vi "Create Coverage Report - With Custom Time Stamp - Reports Same Time.vi"() -> ()   [LabVIEW 2017, in "Cobertura.Tests.lvlib"]
uses:
  Cobertura.Tests.lvlib
  Fake Code Coverage/Fake Code Coverage.lvclass
  C:/Users/pasca/Projects/Home/lvunit/CodeCoverage/CodeCoverage.lvclass
  Fake Code Inspector/Fake Code Inspector.lvclass
  C:/Users/pasca/Projects/Home/lvunit/Cobertura/Code Inspector Base/Code Inspector Base.lvclass
  Fake Project Inspector/Fake Project Inspector.lvclass
  C:/Users/pasca/Projects/Home/lvunit/Cobertura/Project Inspector Base/Project Inspector Base.lvclass
  Cobertura/Coverage/Coverage.lvclass/Coverage.ctl
  Cobertura/Coverage/Read Timestamp.vi
  Cobertura/Cobertura.lvlib
  Cobertura/Coverage/Coverage.lvclass
  <vilib>/PNR/Transparent Assertions/Transparent Assertions/Transparent Assertions.lvlib
panel:
  out "error out":errorcluster
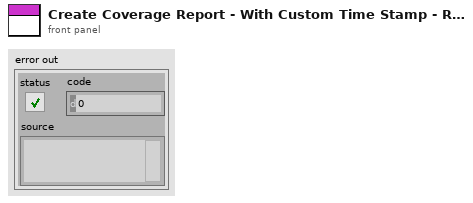
[diagram p1: front panel]
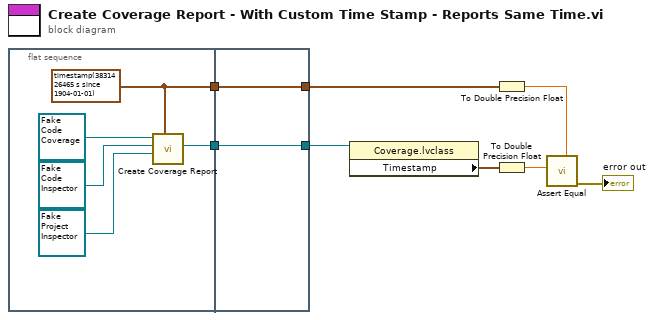
[diagram p0: block diagram]
diagram:
  n1 = flat-sequence {
    tunnel: [w10] -> w7
    tunnel: [w9] -> w2
    tunnel: [w15] -> w8
    tunnel: w7 -> [w15]
    tunnel: [w14] -> w3
    tunnel: w2 -> [w14]
    frame #0 {
      w9 = timestamp(3831426465.529049 s since 1904-01-01) ("Time Stamp (Now)")
      n2 = call "Create Coverage Report.vi"("Time Stamp (Now)"=w9, "Project Inspector"=refnum<class "Fake Project Inspector.lvclass"> refnum ("Cobertura.Tests.lvlib:Fake Project Inspector.lvclass"), "Code Inspector"=refnum<class "Fake Code Inspector.lvclass"> refnum ("Cobertura.Tests.lvlib:Fake Code Inspector.lvclass"), "CodeCoverage in"=refnum<class "Fake Code Coverage.lvclass"> refnum ("Cobertura.Tests.lvlib:Fake Code Coverage.lvclass")) -> ("Coverage"=w10:refnum<class "Coverage.lvclass">)  [unwired: 6 in, 1 out]
    }
    frame #1 {
    }
  }
  n3 = property class="Coverage.lvclass"(reference=w8) -> ("Timestamp"=w6:timestamp)  [unwired: 1 in, 2 out]
  n4 = To Double Precision Float(number=w3) -> (double precision float=w1:dbl)
  n5 = To Double Precision Float(number=w6) -> (double precision float=w5:dbl)
  n6 = call <vilib>:"Assert Equal.vi"("Expected"=w1, "Actual"=w5) -> ("error out"=→"error out":errorcluster)  [unwired: 9 in]
